vi "Add Tag.vi"(5 "Name (Optional)":string, 7 "ID":u32, 8 "error in (no error)":errorcluster, 10 "Tag Value":refnum<class "Basic Type.lvclass">, 11 "Message in":refnum<class "Raw Message.lvclass">) -> (0 "error out":errorcluster, 3 "Message out":refnum<class "Raw Message.lvclass">)   [LabVIEW 2020, in "Protobuf RAW.lvlib" / "Raw Message.lvclass"]
uses:
  Raw Message.lvclass
  Tag/Basic Type.lvclass
  Raw Message.lvclass/Raw Message.ctl
  <vilib>/Utility/miscctls.llb/LVMapReplaceAction.ctl
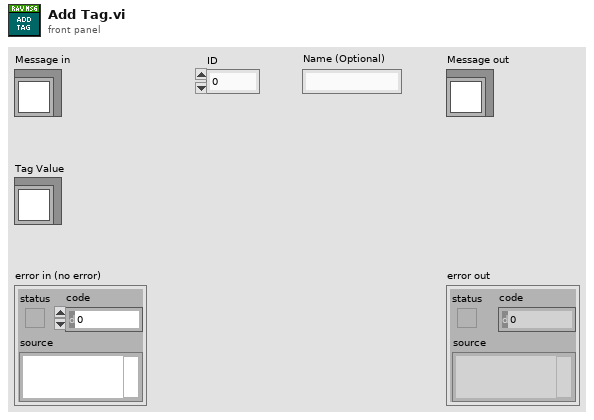
[diagram p1: front panel]
types:
  T1 = typedef "LVMapReplaceAction.ctl" = enum32{"Modify Entry only if found", "Add or Modify Entry", "Delete Entry"}
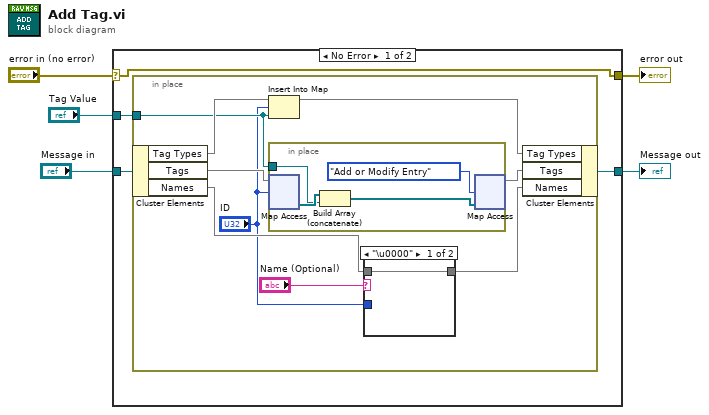
[diagram p0: block diagram]
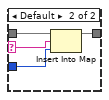
[diagram p2: hidden frame]
diagram:
  n1 = case shown="No Error" "error in (no error)" {
    selector: "error in (no error)" -> [w8 w29]
    tunnel: [w8 w29] -> w4
    tunnel: [w7 w28] -> w2
    tunnel: "Message in" -> [w9 w28]
    tunnel: "Tag Value" -> [w6 _]
    frame No Error {
      n2 = in-place {
        in-place-border: w6 -> [w14]
        n3 = in-place-cluster #1(w9) -> ("Tag Types"=w18:map{u32, refnum<class "Basic Type.lvclass">}, "Tags"=w16:map{u32, refnum<class "Basic Type.lvclass">[]}, "Names"=w13:map{string, u32})
        n4 = Insert Into Map(map in=w18, key="ID", value=w14) -> (map out=w17:map{u32, refnum<class "Basic Type.lvclass">})  [unwired: 2 out]
        n5 = in-place {
          in-place-border: w14 -> [w25]
          n6 = in-place-map #2(w16, "ID") -> (w27:refnum<class "Basic Type.lvclass">[])  [unwired: 1 in, 1 out]
          n7 = Build Array (concatenate)(w27, w25) -> (w26:refnum<class "Basic Type.lvclass">[])
          n8 = in-place-map #2(w26, LVMapReplaceAction."Add or Modify Entry" ("action")) -> (w15:map{u32, refnum<class "Basic Type.lvclass">[]})  [unwired: 2 out]
        }
        n9 = case shown="\"\"" "Name (Optional)" {
          selector: "Name (Optional)" -> [_ w21]
          tunnel: w13 -> [w19 w23]
          tunnel: [w19 w22] -> w12
          tunnel: "ID" -> [_ w20]
          frame "\u0000" {
          }
          frame Default {
            n10 = Insert Into Map(map in=w23, key=w21, value=w20) -> (map out=w22:map{string, u32})  [unwired: 2 out]
          }
        }
        n11 = in-place-cluster #1("Tag Types"=w17, "Tags"=w15, "Names"=w12) -> (w7:refnum<class "Raw Message.lvclass">)
      }
    }
    frame Error {
    }
  }
  "error out" <- w4
  "Message out" <- w2
